vi "Write U8 Array.vi"(8 "error in":errorcluster, 9 "Cluster BLOB in":u8[](array[numeric]), 10 "register offset":u32, 11 "session in":u32) -> (0 "error out":errorcluster, 3 "session out":u32)   [LabVIEW 2018, in "Scalar IO Operations.lvlib"]
uses:
  Scalar IO Operations.lvlib
  NiFpga.dll
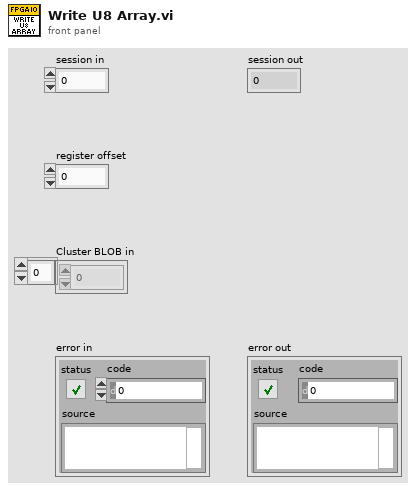
[diagram p1: front panel]
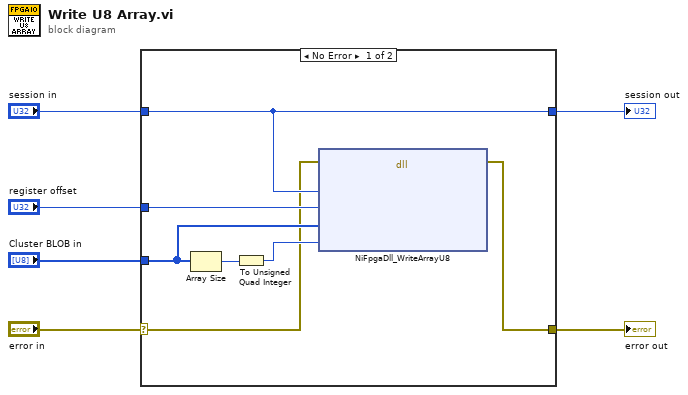
[diagram p0: block diagram]
diagram:
  n1 = case shown="No Error" "error in" {
    selector: "error in" -> [w8 w15]
    tunnel: "session in" -> [w13 w14]
    tunnel: [w7 w15] -> w5
    tunnel: "register offset" -> [w12 _]
    tunnel: [w13 w14] -> w2
    tunnel: "Cluster BLOB in" -> [w11 _]
    frame No Error {
      n2 = Array Size(array=w11) -> (size(s)=w10:i32)
      n3 = To Unsigned Quad Integer(1:w10) -> (0:w9:u64)
      n4 = dll-call lib="NiFpga.*" fn="NiFpgaDll_WriteArrayU8"(error in=w8, "session"=w13, "offset"=w12, "data"=w11, "count"=w9) -> (error out=w7:errorcluster)  [unwired: 7 in, 1 out]
    }
    frame Error {
    }
  }
  "error out" <- w5
  "session out" <- w2
